vi "Error Query Multiple.vi"(0 "VISA resource name":refnum<visa-resource-name>, 11 "error in (no error)":errorcluster) -> (4 "VISA resource name out":refnum<visa-resource-name>, 8 "Error":i32[](array[numeric]), 10 "Error Message":string, 15 "error out":errorcluster)   [LabVIEW 2013, in "Yokogawa PZ4000.lvlib"]
doc: "This VI reads the error queue from the instrument. It expects to see errors in SCPI format (#,\"error message\"). It continues to read from the error queue until it reads a 0, \"No error\"."
uses:
  Yokogawa PZ4000.lvlib
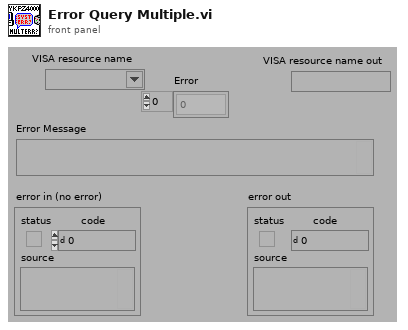
[diagram p1: front panel]
types:
  T1 = cluster{"Status":bool, "Error":i32, "source":string}
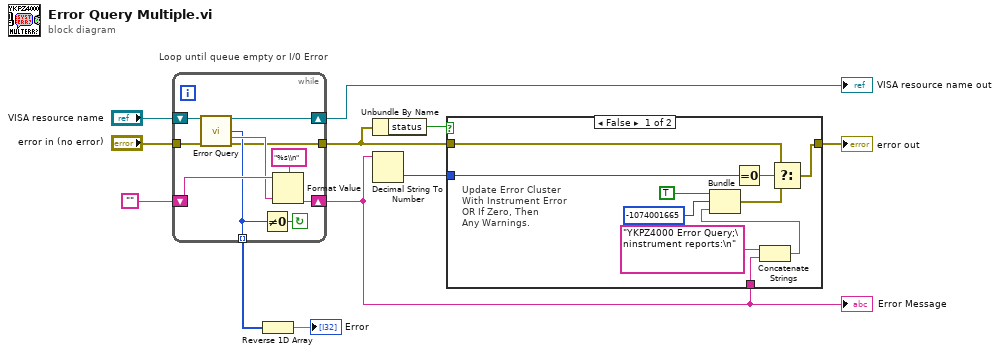
[diagram p0: block diagram]
diagram:
  # "Loop until queue empty or I/0 Error"
  n1 = while {
    tunnel: "error in (no error)" -> [w12]
    tunnel: [w15] -> w7 mode=indexing
    tunnel: [w13] -> w4
    shift-left: "VISA resource name" -> [w14]
    shift-right: [w21] -> w10
    shift-left: "" -> [w18]
    shift-right: [w20] -> w1
    stop <- w16 continue-if-true
    n2 = call "Error Query.vi"("VISA resource name"=w14, "error in (no error)"=w12) -> ("VISA resource name out"=w21:refnum<visa-resource-name>, "Error"=w15:i32, "Error Message"=w17:string, "error out"=w13:errorcluster)  [unwired: 10 in]
    n3 = Not Equal To 0?(x=w15) -> (x != 0?=w16:bool)
    n4 = Format Value(string ("")=w18, format string="%s\\n", value (0)=w17) -> (output string=w20:string)
  }
  "Error Message" <- w1
  "VISA resource name out" <- w10
  n5 = Reverse 1D Array(array=w7) -> (reversed array=→"Error":i32[])
  n6 = Unbundle By Name(w4) -> ("status"=w5:bool)
  n7 = Decimal String To Number(string=w1) -> (number=w3:i32)  [unwired: 2 in, 1 out]
  n8 = case shown="False" w5 {
    tunnel: w3 -> [w22 _]
    tunnel: [w25 w32] -> w2
    tunnel: w4 -> [w24 w32]
    tunnel: w1 -> [w31 _]
    frame False {
      # "Update Error Cluster\nWith Instrument Error \nOR If Zero, Then \nAny Warnings."
      n9 = Equal To 0?(x=w22) -> (x = 0?=w26:bool)
      n10 = Concatenate Strings("YKPZ4000 Error Query;\ninstrument reports:\n" ("Source"), w31) -> (w28:string)
      n11 = Bundle("Status"=TRUE, "Error"=-1074001665, w28) -> (w23:cluster{"Status":bool, "Error":i32, string})  [unwired: 1 in]
      n12 = Select(t=w24, s=w26, f=w23) -> (s? t:f=w25:T1)
    }
    frame True {
      # "IO Error"
    }
  }
  "error out" <- w2
